vi "dfd_Get Specified Subband Filters.vi"(8 "error in":errorcluster, 10 "subband index":i32[](array[numeric]), 11 "bank":T6 {"mBank_Type" items=["Uniform", "Non-Uniform"]; "mBank_Filters"."mMRate_SumWl" min=1 max=32 step=1; "mBank_Filters"."mMRate_InputIwl" min=1 max=32 step=1; "mBank_Filters"."mMRate_GainWl" min=1 max=32 step=1; "mBank_Filters"."mMRate_OutputWl" min=1 max=32 step=1; "mBank_Filters"."mMRate_InputWl" min=1 max=32 step=1; "mBank_Filters"."mMRate_CoefWl" min=1 max=32 step=1; "mBank_Filters"."mMRate_Mode" items=["Default"=-1, "No Rate Change"=0, "Interpolation"=1, "Decimation"=2, "Interpolated"=3, "Rational"=4]}) -> (0 "error out":errorcluster, 2 "subband filters":T1[](array[typedef]) {"mMRate_SumWl" min=1 max=32 step=1; "mMRate_InputIwl" min=1 max=32 step=1; "mMRate_GainWl" min=1 max=32 step=1; "mMRate_OutputWl" min=1 max=32 step=1; "mMRate_InputWl" min=1 max=32 step=1; "mMRate_CoefWl" min=1 max=32 step=1; "mMRate_Mode" items=["Default"=-1, "No Rate Change"=0, "Interpolation"=1, "Decimation"=2, "Interpolated"=3, "Rational"=4]})   [LabVIEW 2017, in "NI_DigFilter_FilterBank.lvlib"]
uses:
  <vilib>/addons/Digital Filter Design/NI_DigFilter_FilterBank.lvlib
  <vilib>/addons/Digital Filter Design/FilterBank.llb/Object/DFD Bank Obj.ctl
  <vilib>/addons/Digital Filter Design/_Objects.llb/DFD Multirate Filter Obj.ctl
  <vilib>/addons/Digital Filter Design/_Objects.llb/DFD Multirate Mode.ctl
  <vilib>/addons/Digital Filter Design/_Objects.llb/DFD Coef Norm Type.ctl
  <vilib>/addons/Digital Filter Design/_Objects.llb/DFD Round-off Mode.ctl
  <vilib>/addons/Digital Filter Design/_Objects.llb/DFD FXP MRate Multiply Mode.ctl
  <vilib>/addons/Digital Filter Design/FilterBank.llb/Object/DFD Filter Bank Processing Method.ctl
  <vilib>/addons/Digital Filter Design/FilterBank.llb/Object/DFD Filter Bank Type.ctl
  <vilib>/addons/Digital Filter Design/_Misc.llb/dfd_Error Handlers (Single).vi
  <vilib>/addons/Digital Filter Design/NI_DigFilterLicensed.lvlib
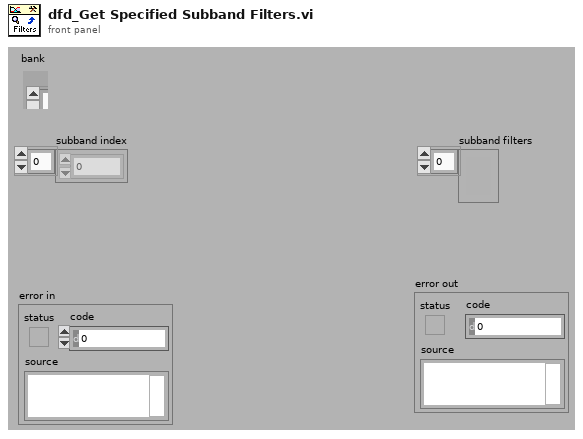
[diagram p1: front panel]
types:
  T1 = typedef "NI_DigFilterLicensed.lvlib/DFD Multirate Filter Obj.ctl" = cluster{"mMRate_Structure":enum16{"CIC", "FIR", "IIR", "Lattice"}, "mMRate_Mode":T2, "mMRate_Factor":i32, "mMRate_FIRParams":cluster{"mMRate_FIR_H":dbl[], "mMRate_FIR_IsNyquist?":bool, "mMRate_FIR_IsSymmetric?":bool}, "mMRate_CICParams":cluster{"mMRate_CIC_#Stage":i32, "mMRate_CIC_Lag":i32, "mMRate_CIC_Type":enum16{"Lowpass", "Highpass"}}, "mMRate_Order":i32, "mMRate_Version":string, "mMRate_Comments":string, "mMRate_RationalFactor":cluster{"mMRate_L":i32, "mMRate_M":i32}, "mMRate_Fs":dbl, "mMRate_Quantized?":bool, "mMRate_QFilterGain":dbl, "mMRate_CoefWl":i16, "mMRate_Scaling":cluster{"mMRate_ScaleByPowerOf2?":bool, "mMRate_ScaleType":T3}, "mMRate_InputWl":i16, "mMRate_OutputWl":i16, "mMRate_OutputMode":T4, "mMRate_MultMode":T5, "mMRate_BitPruning":bool, "mMRate_GainWl":i16, "mMRate_OutputFwl":i16, "mMRate_SumIwl":i16, "mMRate_InputIwl ":i16, "mMRate_SumWl":i16, "mMRate_CoefIwl":i16}
  T2 = typedef "NI_DigFilterLicensed.lvlib/DFD Multirate Mode.ctl" = i16
  T3 = typedef "NI_DigFilterLicensed.lvlib/DFD Coef Norm Type.ctl" = enum16{"No Norm", "Time Domain 1-Norm", "Time Domain 2-Norm", "Time Domain Inf-Norm"}
  T4 = typedef "NI_DigFilterLicensed.lvlib/DFD Round-off Mode.ctl" = enum16{"Nearest", "Truncation"}
  T5 = typedef "NI_DigFilterLicensed.lvlib/DFD FXP MRate Multiply Mode.ctl" = enum16{"Truncated", "Full"}
  T6 = typedef "NI_DigFilter_FilterBank.lvlib/DFD Bank Obj.ctl" = cluster{"mBank_Filters":T1[], " mBank_#Bands":i32, "mBank_ProcMethod":T7, "mBank_Coeffs":dbl[], "mBank_Gain":dbl, "mBank_Type":T8}
  T7 = typedef "NI_DigFilter_FilterBank.lvlib/DFD Filter Bank Processing Method.ctl" = enum16{"General", "2-Band QMF Lattice", "Cosine-Modulated"}
  T8 = typedef "NI_DigFilter_FilterBank.lvlib/DFD Filter Bank Type.ctl" = u16
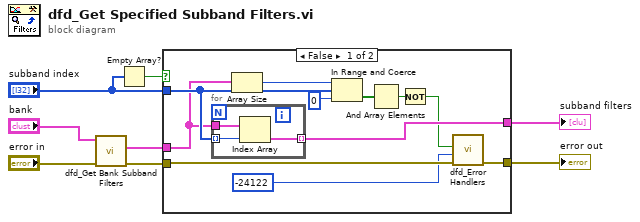
[diagram p0: block diagram]
diagram:
  n1 = call <vilib>:"dfd_Get Bank Subband Filters.vi"("error in (no error)"="error in", "bank in"="bank") -> ("error out"=w4:errorcluster, "subband filters"=w2:T1[])  [unwired: 6 in, 2 out]
  n2 = Empty Array?(array="subband index") -> (empty?=w1:bool)
  n3 = case shown="False" w1 {
    tunnel: w2 -> [w17 w24]
    tunnel: [w19 w24] -> w5
    tunnel: "subband index" -> [w18 _]
    tunnel: w4 -> [w12 w23]
    tunnel: [w13 w23] -> w6
    frame False {
      n4 = for {
        tunnel: w17 -> [w22]
        tunnel: w18 -> [w21] mode=indexing
        tunnel: [w20] -> w19 mode=indexing
        n5 = Index Array(array=w22, index=w21) -> (element=w20:T1)
      }
      n6 = Array Size(array=w17) -> (size(s)=w16:i32)
      n7 = In Range and Coerce(upper limit=w16, x=w18, lower limit=0) -> (In Range?=w14:bool[])  [unwired: 1 out]
      n8 = And Array Elements(Boolean array=w14) -> (logical AND=w10:bool)
      n9 = Not(x=w10) -> (.not. x?=w9:bool)
      n10 = call-poly <vilib>:"dfd_Error Handlers.vi"("error in (no error)"=w12, "error code"=-24122 ("ERR_INVALID_SUBBAND_INDEX"), "condition failed?"=w9) -> ("error out"=w13:errorcluster)  [unwired: 8 in]
    }
    frame True {
    }
  }
  "error out" <- w6
  "subband filters" <- w5
